vi "Demo_Copy.vi"() -> ()   [LabVIEW 2018]
uses:
  <vilib>/Hampel Software Engineering/S7NetCom/Source/Controls/S7_Start_Address.ctl
  <vilib>/Hampel Software Engineering/S7NetCom/Source/Controls/S7_Memory_Area.ctl
  <vilib>/Hampel Software Engineering/S7NetCom/Source/Controls/S7_Variable_Type.ctl
  <vilib>/Hampel Software Engineering/S7NetCom/Source/API/Write Data - Boolean (Scalar).vi
  <vilib>/Hampel Software Engineering/S7NetCom/Source/API/Write Data - String.vi
  <vilib>/Hampel Software Engineering/S7NetCom/Source/API/Write Data - DTL (Scalar).vi
  <vilib>/Hampel Software Engineering/S7NetCom/Source/API/Write Data - Siemens Date & Time (Scalar).vi
  <vilib>/Hampel Software Engineering/S7NetCom/Source/API/Write Data - Byte (Scalar).vi
  <vilib>/Hampel Software Engineering/S7NetCom/Source/API/Write Data - Word (Scalar).vi
  <vilib>/Hampel Software Engineering/S7NetCom/Source/API/Write Data - Real (Scalar).vi
  <vilib>/Hampel Software Engineering/S7NetCom/Source/API/Write Data - Real (1D Array).vi
  <vilib>/Hampel Software Engineering/S7NetCom/Source/API/Read Data - Boolean (Scalar).vi
  <vilib>/Hampel Software Engineering/S7NetCom/Source/API/Read Data - String.vi
  <vilib>/Hampel Software Engineering/S7NetCom/Source/API/Read Data - DTL (Scalar).vi
  <vilib>/Hampel Software Engineering/S7NetCom/Source/API/Read Data - Siemens Date&Time (Scalar).vi
  <vilib>/Hampel Software Engineering/S7NetCom/Source/API/Read Data - Byte (Scalar).vi
  <vilib>/Hampel Software Engineering/S7NetCom/Source/API/Read Data - Word (Scalar).vi
  <vilib>/Hampel Software Engineering/S7NetCom/Source/API/Read Data - Real (Scalar).vi
  <vilib>/Hampel Software Engineering/S7NetCom/Source/API/Read Data - Real (1D Array).vi
  <vilib>/Hampel Software Engineering/S7NetCom/Source/S7NetCom.lvclass
panel:
  out "time(ms)":u32
  in  "Tab Control TX":T1(tab)
  in  "TX Data":u32[](array[numeric])
  in  "Btn_WriteRaw":bool
  in  "Btn_WriteBOOL":bool
  in  "Boolean Value (TX)":bool
  out "Boolean Value (RX)":bool
  in  "Btn_ReadBOOL":bool
  in  "Btn_WriteBYTE":bool
  in  "Byte Value (TX)":u8
  out "Byte Value (RX)":u8
  in  "Btn_ReadBYTE":bool
  in  "Btn_WriteWORD":bool
  in  "Word Value (TX)":u16
  out "Word Value (RX)":u16
  in  "Btn_ReadWORD":bool
  in  "Btn_WriteREAL":bool
  in  "Real Value (TX)":sgl
  out "Real Value (RX)":sgl
  in  "Btn_ReadREAL":bool
  in  "Real Values (TX)":sgl[](array[numeric])
  in  "Btn_WriteREALArray":bool
  in  "Btn_ReadREALArray":bool
  out "Real Values (RX)":sgl[](array[numeric])
  in  "String Read Length":u16
  out "String Value (RX)":string
  in  "String Value (TX)":string
  in  "Btn_WriteSTRING":bool
  in  "Btn_ReadSTRING":bool
  in  "Btn_ReadDTL":bool
  out "DTL Value (RX)":timestamp
  in  "DTL (TX)":timestamp
  in  "Btn_Write DTL":bool
  in  "Date & Time (TX)":timestamp
  in  "Btn_Write D&T":bool
  in  "Btn_ReadD&T":bool
  out "Date&Time Value (RX)":timestamp
  in  "stop":bool
  in  "Count":u16=1 caption="Read Length"
  in  "Start Address":T2
  in  "Data Block #":u16=2
  in  "RAW Var Type":T3=enum."BYTE"
  in  "Memory Area":T4=132 items=["P Area"=128, "I Area"=129, "O Area"=130, "M Area"=131, "DB Area"=132, "Counter"=40, "Timer"=41]
  in  "Bit Offset":u8
  out "Read/Write Error out":errorcluster
  out "U32":i32[](array[numeric])
  out "String":string
  out "Char's":string[](array[string])
  out "Bits (1st byte)":bool[](array[boolean])
  in  "Cont Variable Type":T3=enum."BYTE" caption="Variable Type"
  in  "Cont Memory Area":T4=132 caption="Memory Area" items=["P Area"=128, "I Area"=129, "O Area"=130, "M Area"=131, "DB Area"=132, "Counter"=40, "Timer"=41]
  in  "Cont Start Address":T2 caption="Start Address"
  in  "Cont Read Length":u16=1 caption="Read Length"
  in  "Cont Data Block #":u16=2 caption="Data Block #"
  out "Real (32bit)":sgl
  in  "Cont Bit Offset":u8 caption="Bit Offset"
  out "Seq No":u16
  in  "Cont TO":i32=250
  in  "Rack":u8
  out "Error out":errorcluster caption="Read Continuously Error out"
  in  "IP Address":string
  in  "Port":i32=102
  in  "Slot":u8=1
  in  "Timeout":i32=5000
  # "Connection"
  # "Read Continuously"
  # "Read / Write"
  # "说明：感谢该组织开源库，\n本VI为拷贝自S7NetCom库，通过安装S7NetCom.vip可在安装目录获取该范例。\n粗略测试，一次最多读230个字节，低延时。"
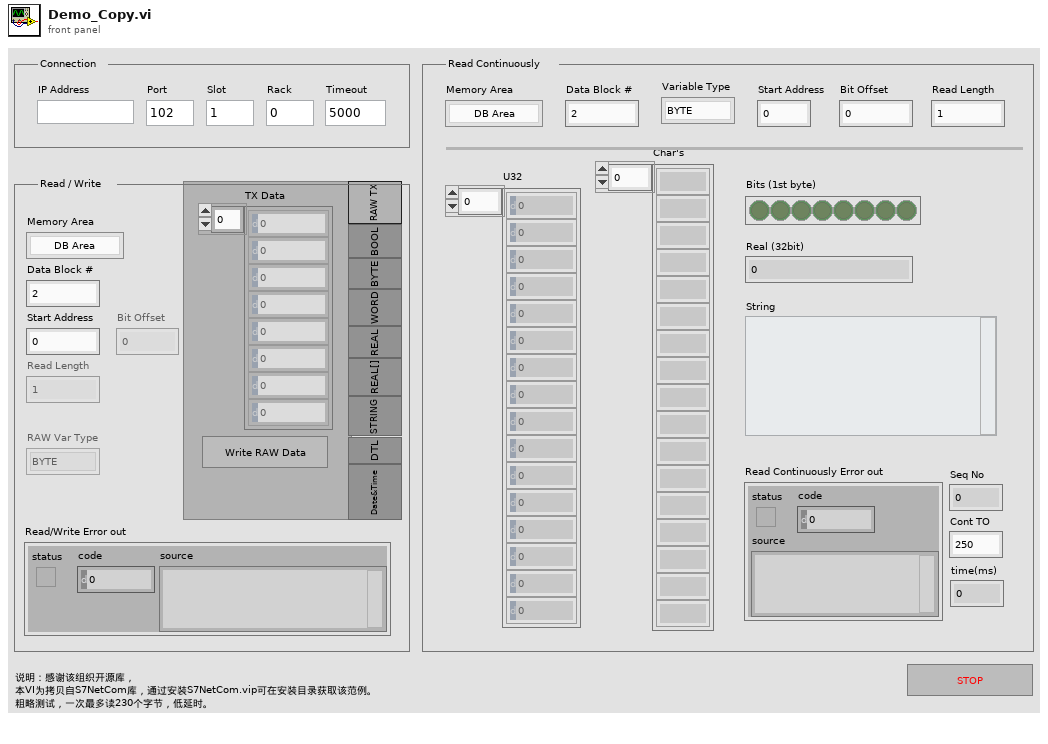
[diagram p1: front panel]
types:
  T1 = enum32{"RAW TX", "BOOL", "BYTE", "WORD", "REAL", "REAL[]", "STRING", "DTL", "Date&Time"}
  T2 = typedef "S7NetCom.lvlib/S7NetCom.lvclass/S7_Start_Address.ctl" = u32
  T3 = typedef "S7NetCom.lvlib/S7NetCom.lvclass/S7_Variable_Type.ctl" = enum8{"---", "BIT", "BYTE", "CHAR", "WORD", "INT", "DWORD", "DINT", "REAL"}
  T4 = typedef "S7NetCom.lvlib/S7NetCom.lvclass/S7_Memory_Area.ctl" = u8
  T5 = enum8{"Enabled", "Disabled", "Disabled and Grayed Out"}
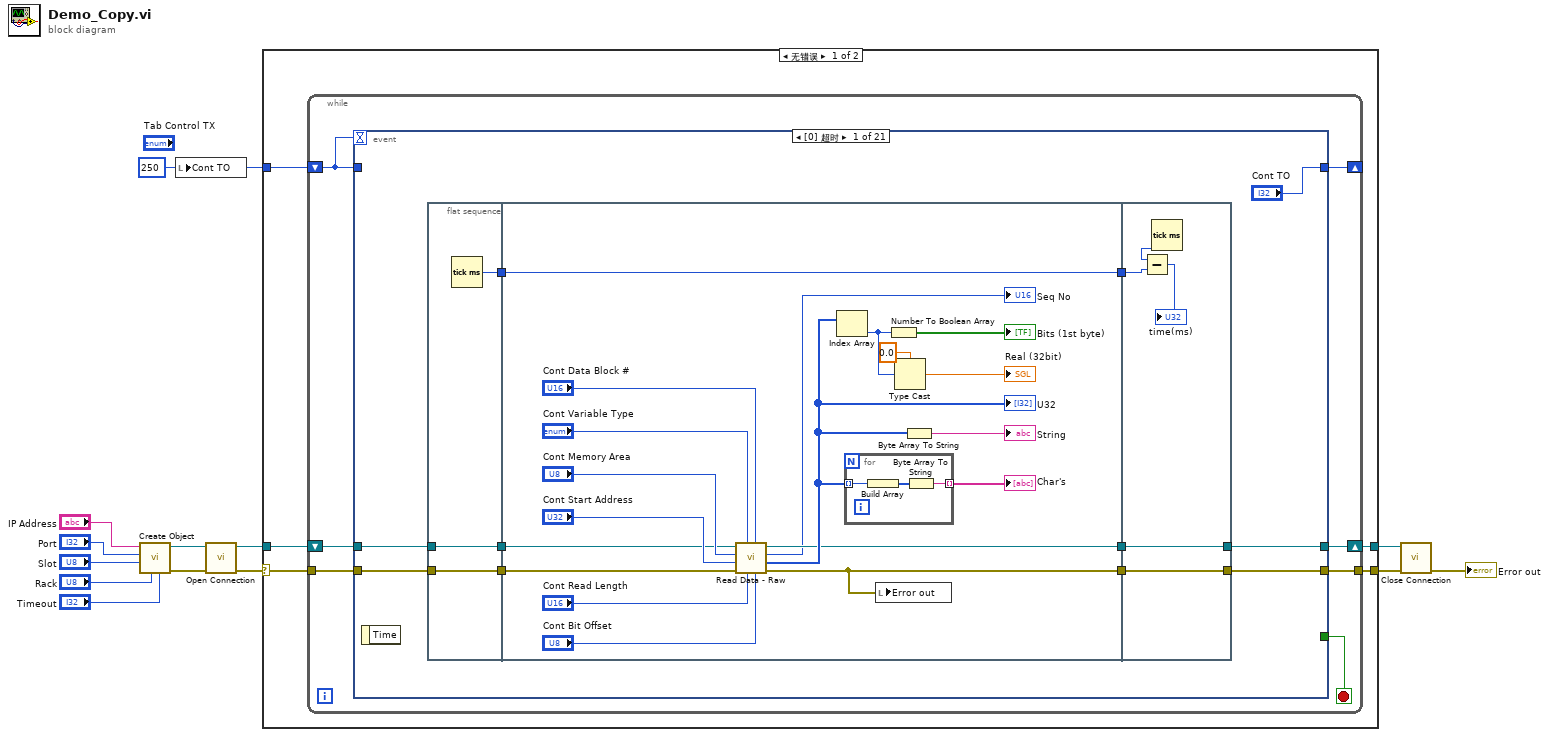
[diagram p0: block diagram]
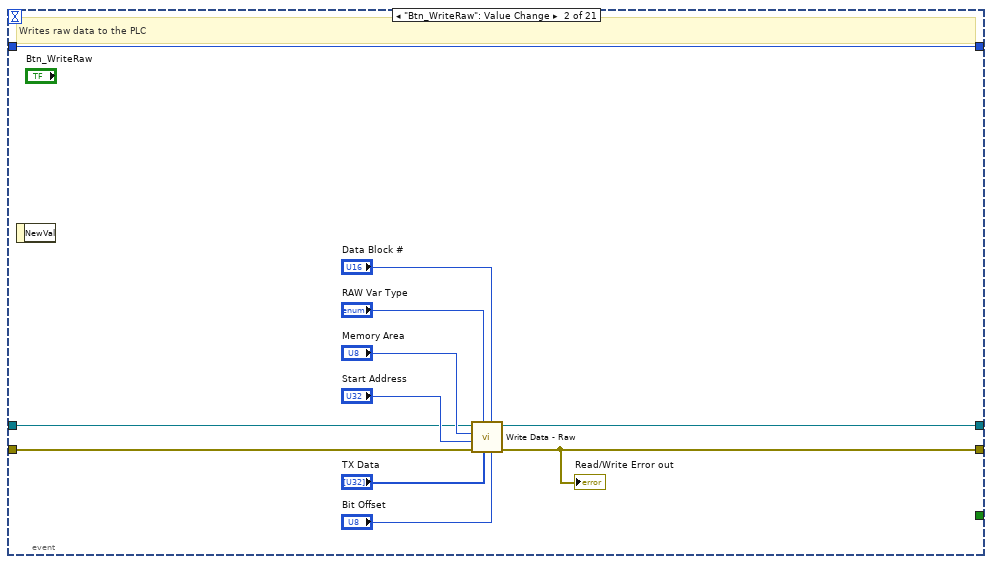
[diagram p2: hidden frame]
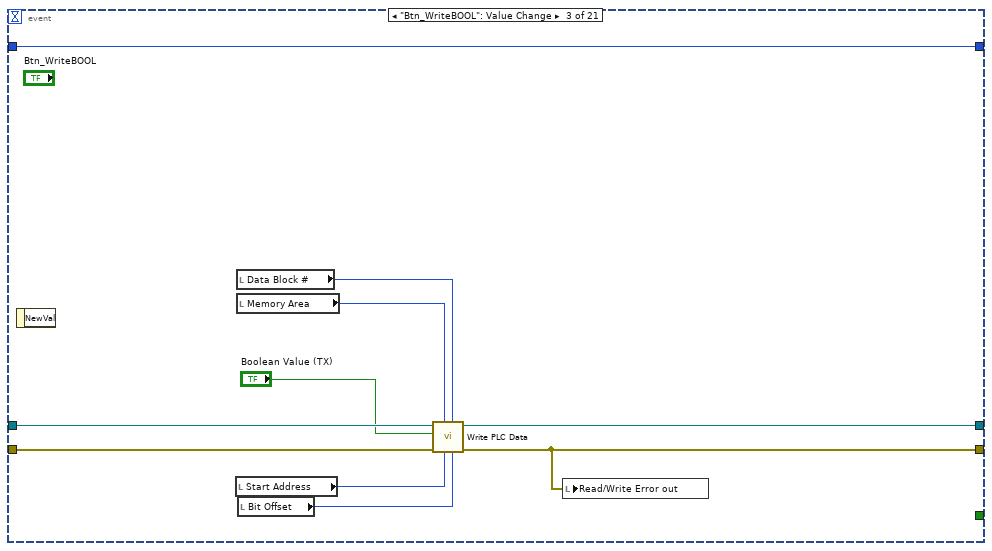
[diagram p3: hidden frame]
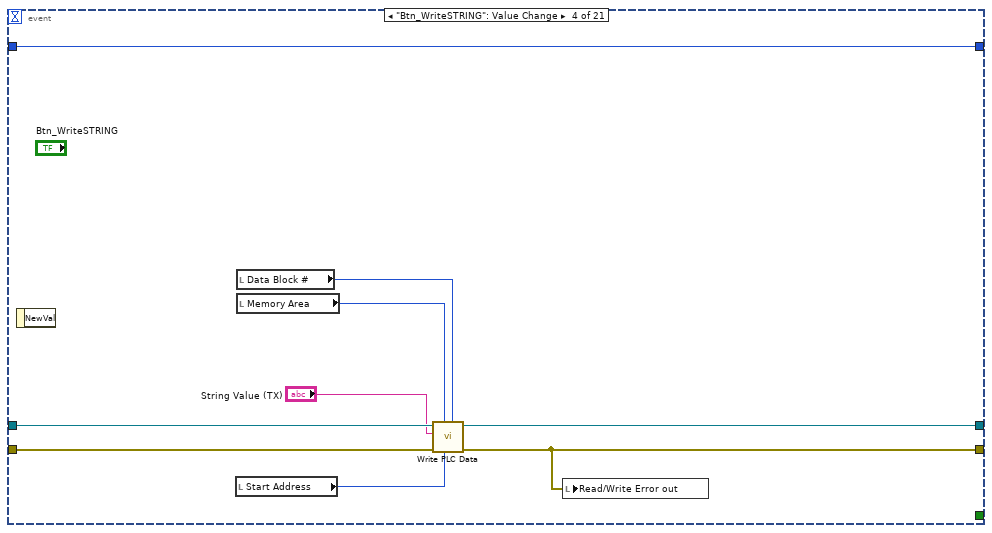
[diagram p4: hidden frame]
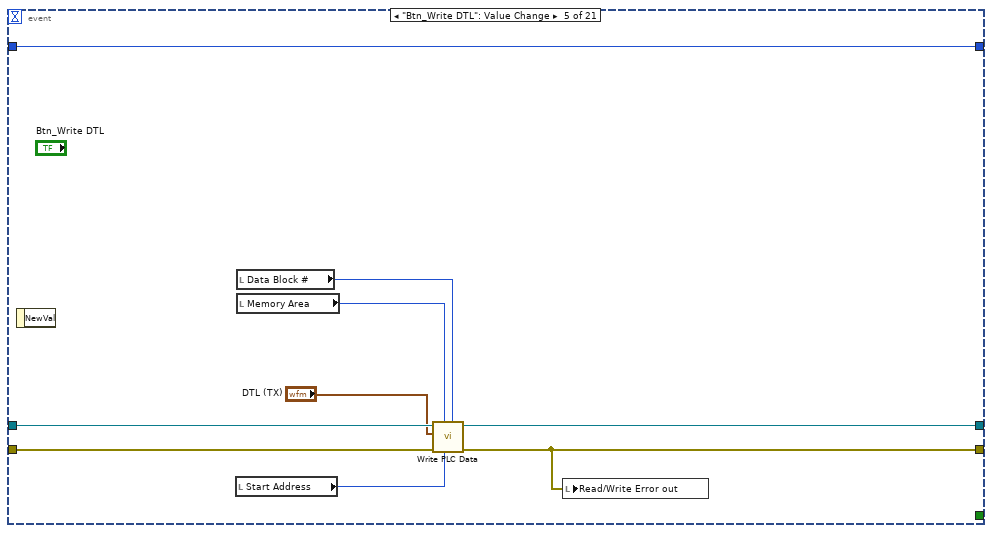
[diagram p5: hidden frame]
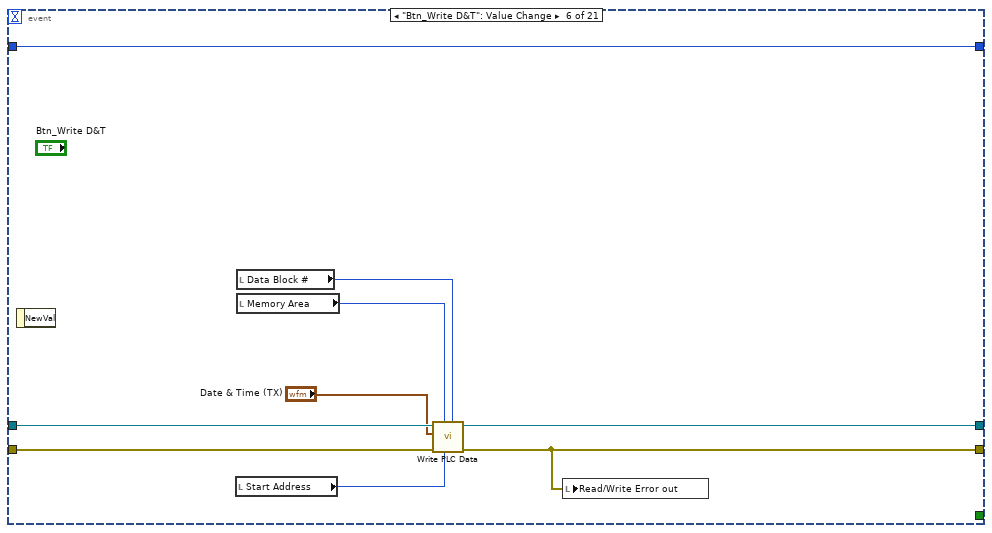
[diagram p6: hidden frame]
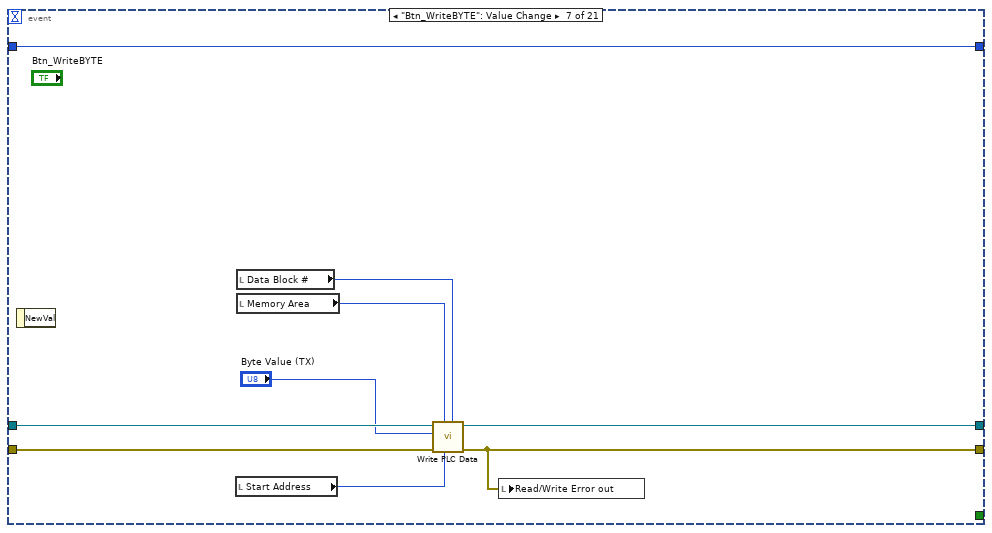
[diagram p7: hidden frame]
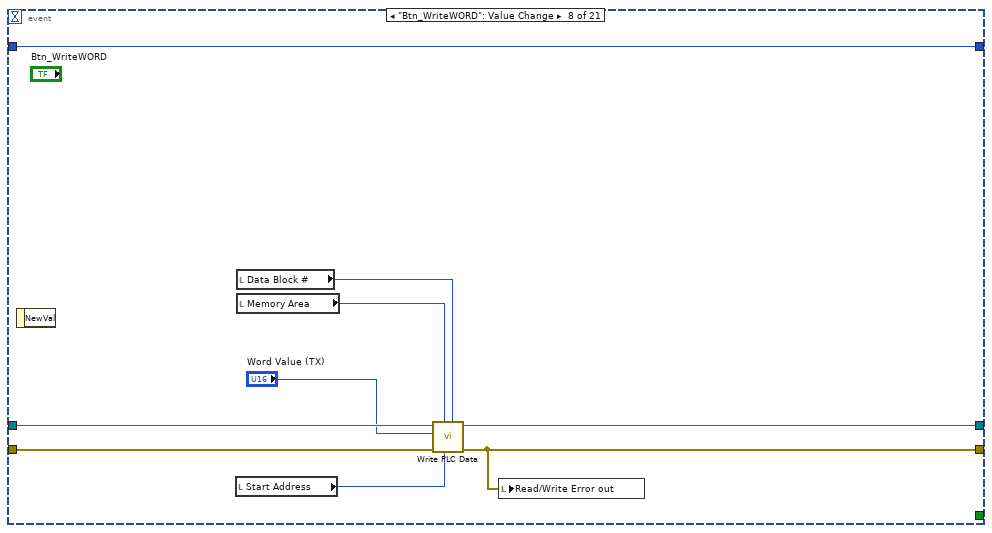
[diagram p8: hidden frame]
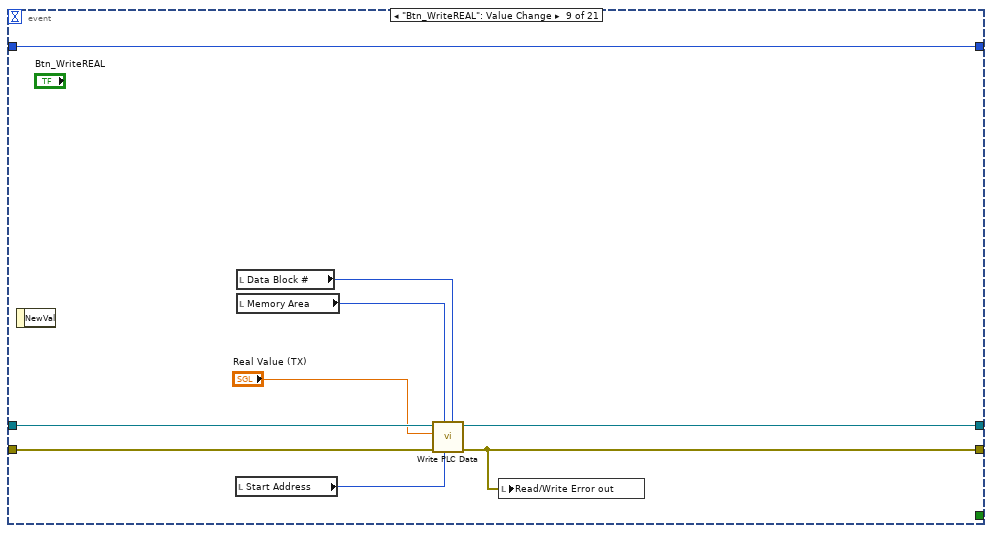
[diagram p9: hidden frame]
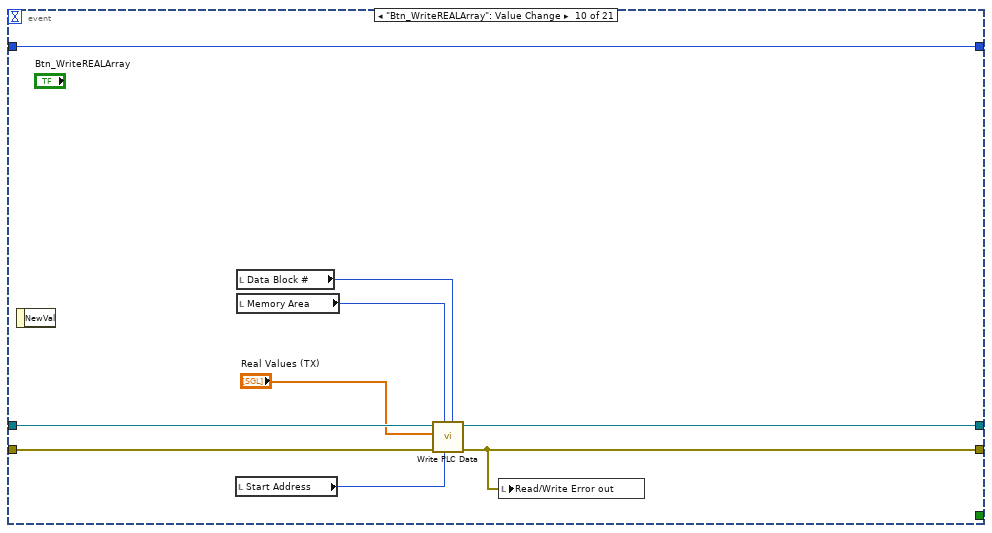
[diagram p10: hidden frame]
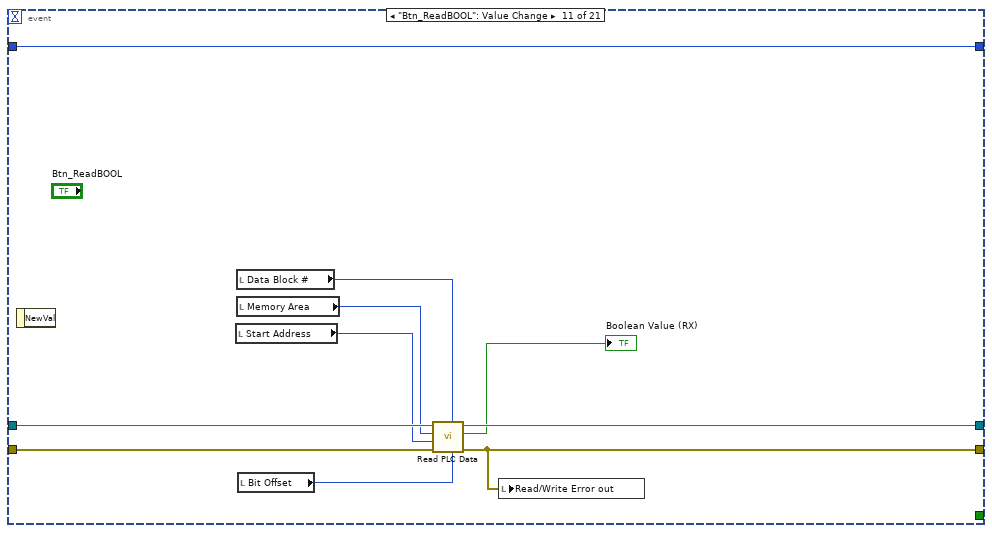
[diagram p11: hidden frame]
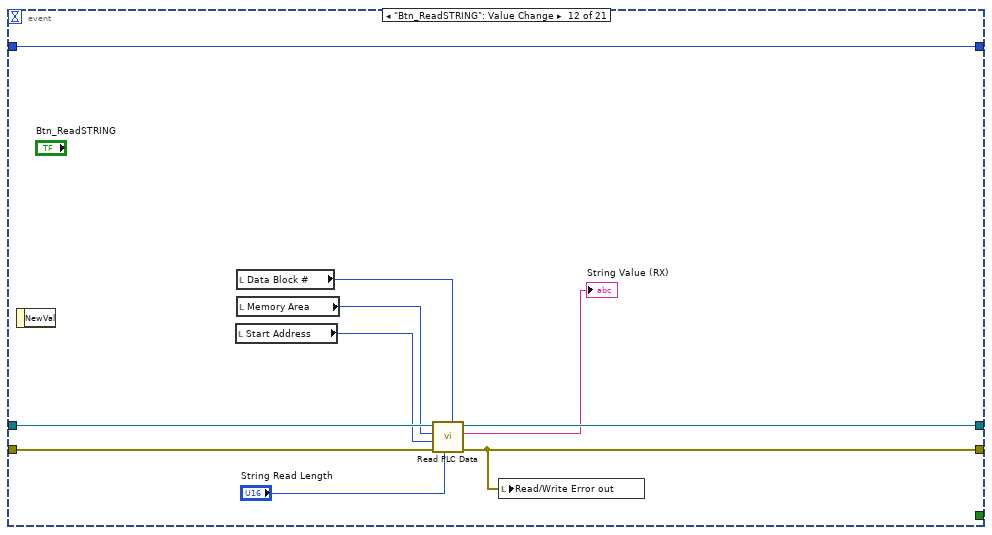
[diagram p12: hidden frame]
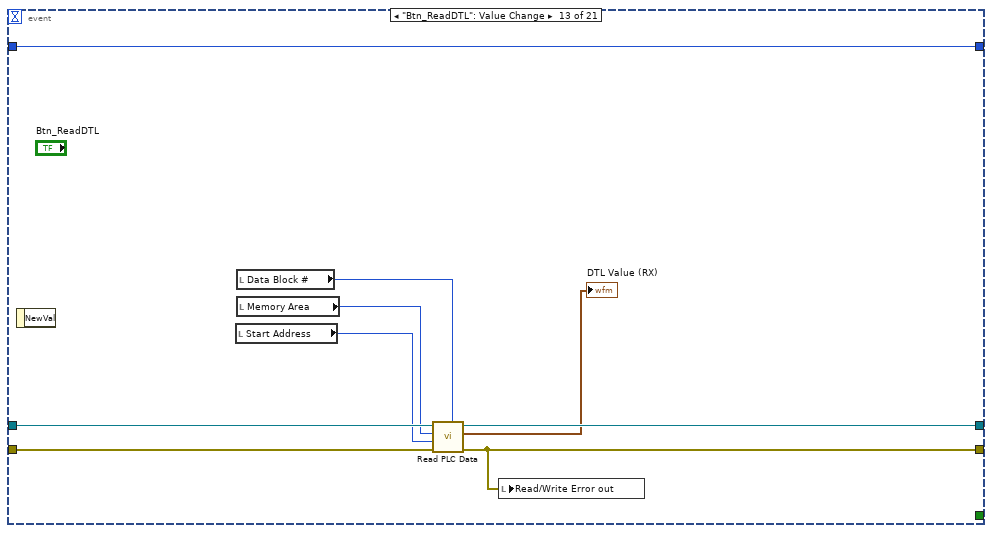
[diagram p13: hidden frame]
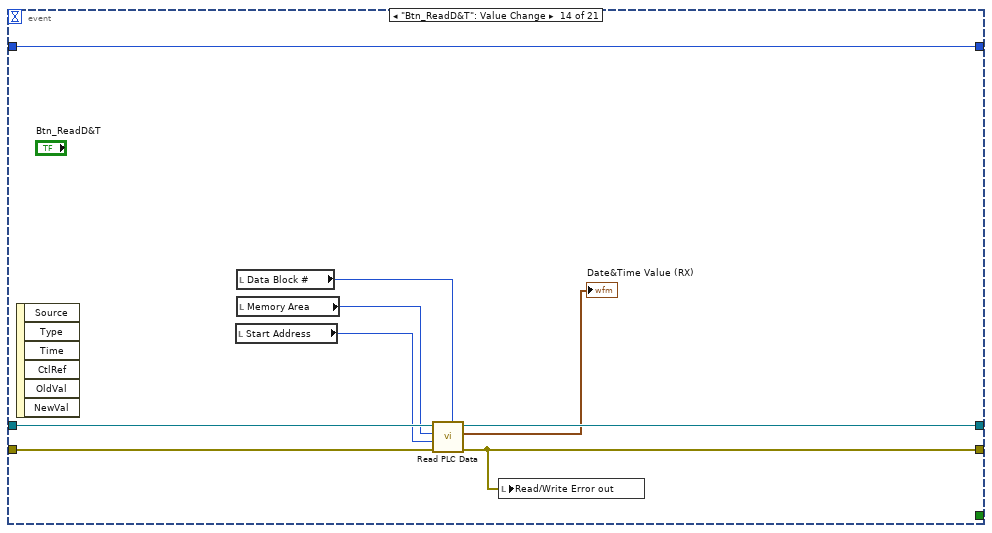
[diagram p14: hidden frame]
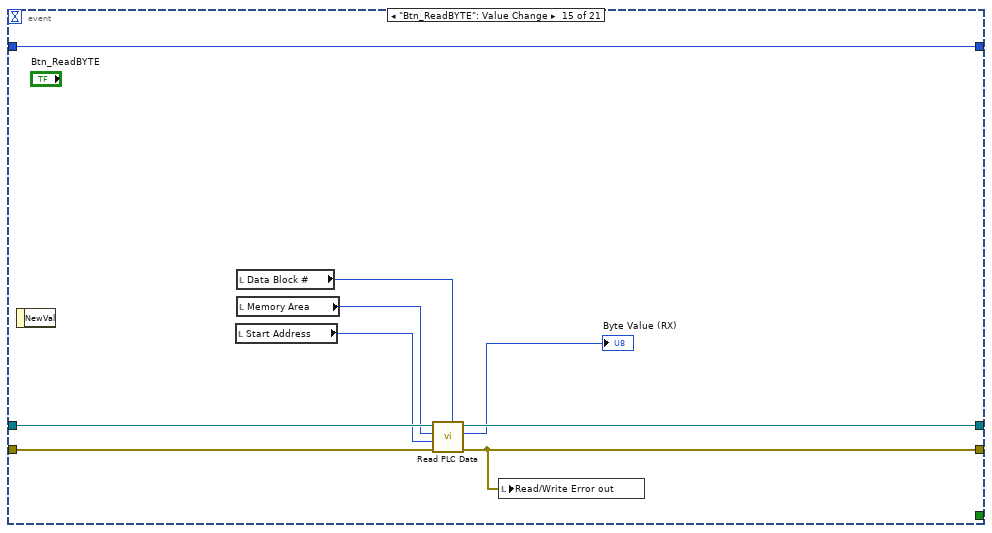
[diagram p15: hidden frame]
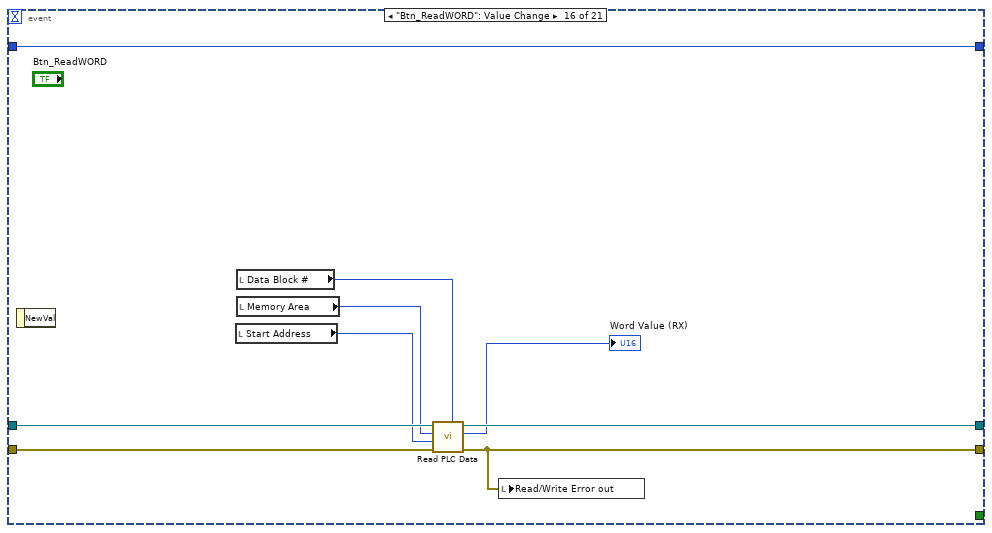
[diagram p16: hidden frame]
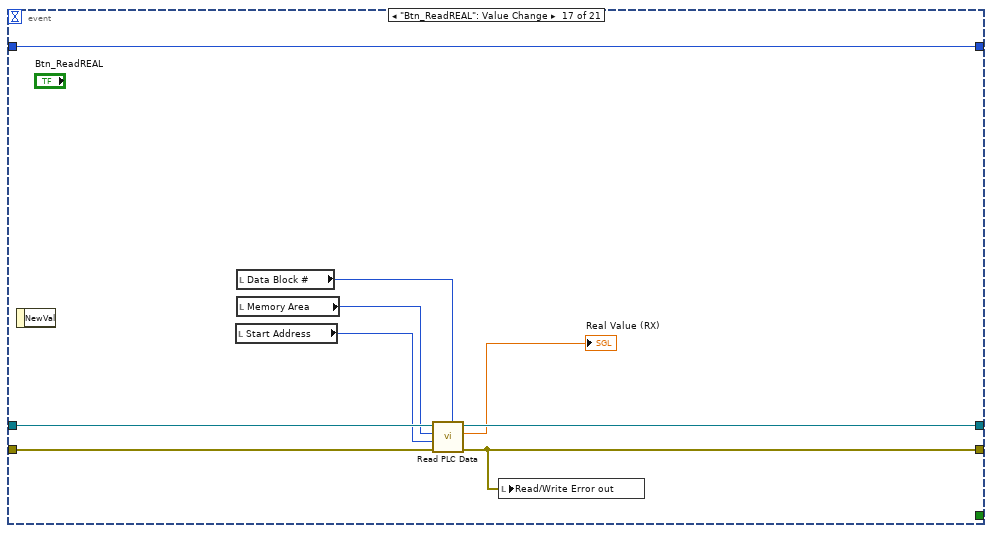
[diagram p17: hidden frame]
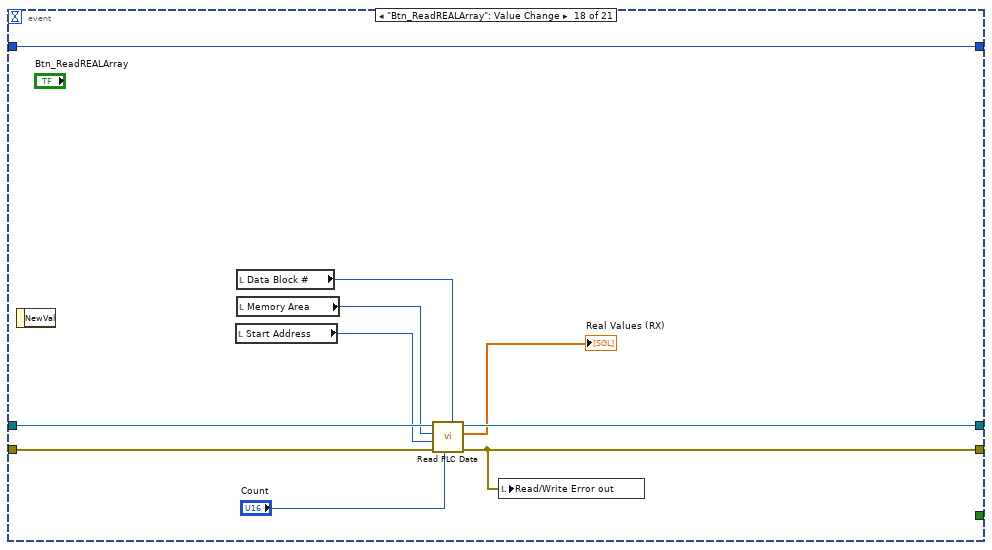
[diagram p18: hidden frame]
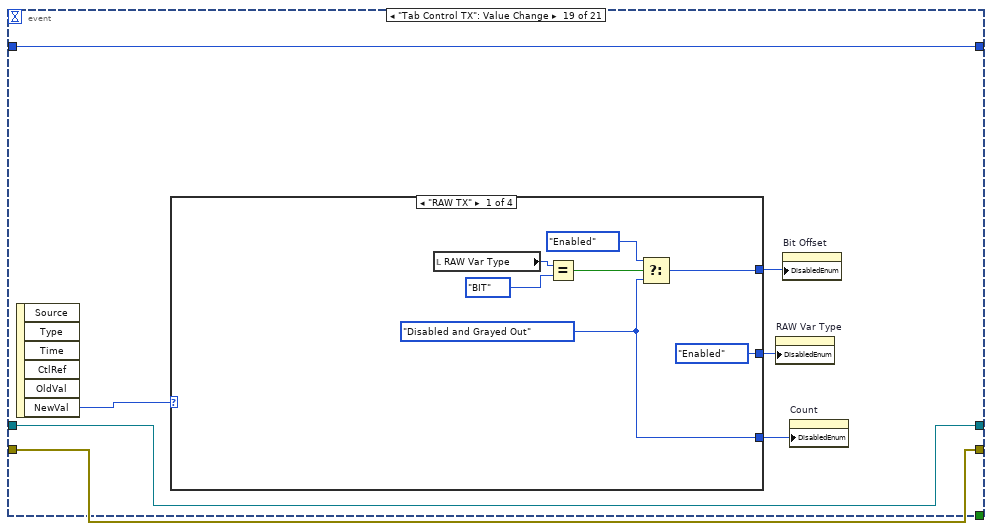
[diagram p19: hidden frame]
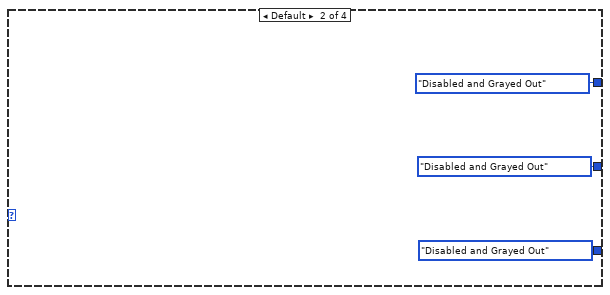
[diagram p20: hidden frame]
diagram:
  w1 = 250
  n1 = call <vilib>:"Create Object.vi"("Timeout"="Timeout", "Rack"="Rack", "Slot"="Slot", "Port"="Port", "IP Address"="IP Address") -> ("error out"=w10:errorcluster, "S7NetCom out"=w13:refnum<class "S7NetCom.lvclass">)  [unwired: 5 in]
  n2 = local write "Cont TO"(w1) -> ()
  n3 = call <vilib>:"Open Connection.vi"("error in"=w10, "S7NetCom in"=w13) -> ("error out"=w9:errorcluster, "S7NetCom out"=w12:refnum<class "S7NetCom.lvclass">)  [unwired: 8 in]
  n4 = case shown="无错误" w9 {
    selector: w9 -> [w15 w259]
    tunnel: w12 -> [w18 w260]
    tunnel: [w17 w260] -> w11
    tunnel: [w16 w259] -> w8
    tunnel: w1 -> [w14 _]
    frame No Error {
      n5 = while {
        shift-right: [w23] -> w17
        shift-left: w18 -> [w25]
        tunnel: [w21] -> w16
        tunnel: w15 -> [w22]
        shift-right: [w19] -> _
        shift-left: w14 -> [w20]
        stop <- w24 stop-if-true
        n6 = event shown="[0] 超时" {
          selector: _ -> [_ _ _ _ _ _ _ _ _ _ _ _ _ _ _ _ _ _ _ _ _]
          dyn-events: _ -> [_ _ _ _ _ _ _ _ _ _ _ _ _ _ _ _ _ _ _ _ _]
          timeout: w20 -> [_ _ _ _ _ _ _ _ _ _ _ _ _ _ _ _ _ _ _ _ _]
          tunnel: w25 -> [w36 w70 w86 w95 w104 w113 w122 w131 w140 w149 w159 w169 w178 w187 w196 w205 w214 w224 w226 w250 w257]
          tunnel: [_ _ _ _ _ _ _ _ _ _ _ _ _ _ _ _ _ _ _ _ w258] -> w24
          tunnel: [w35 w69 w84 w93 w102 w111 w120 w129 w138 w147 w157 w167 w176 w185 w194 w203 w212 w222 w226 w250 w257] -> w23
          tunnel: w22 -> [w33 w71 w87 w96 w105 w114 w123 w132 w141 w150 w160 w170 w179 w188 w197 w206 w215 w225 w227 w251 w256]
          tunnel: [w34 w68 w85 w94 w103 w112 w121 w130 w139 w148 w158 w168 w177 w186 w195 w204 w213 w223 w227 w251 w256] -> w21
          tunnel: w20 -> [_ w67 w78 w89 w98 w107 w115 w124 w133 w142 w151 w163 w172 w181 w189 w198 w207 w216 w232 w252 w255]
          tunnel: ["Cont TO" w67 w78 w89 w98 w107 w115 w124 w133 w142 w151 w163 w172 w181 w189 w198 w207 w216 w232 w252 w255] -> w19
          event Timeout {
            n7 = event-data() -> ()  [unwired: 1 in, 1 out]
            n8 = flat-sequence {
              tunnel: w33 -> [w38]
              tunnel: w36 -> [w39]
              tunnel: [w39] -> w31
              tunnel: [w38] -> w30
              tunnel: [w37] -> w27
              tunnel: w31 -> [w46]
              tunnel: w30 -> [w43]
              tunnel: [w45] -> w29
              tunnel: [w44] -> w28
              tunnel: w27 -> [w40]
              tunnel: [w40] -> w26
              tunnel: [w65] -> w34
              tunnel: [w66] -> w35
              tunnel: w29 -> [w66]
              tunnel: w28 -> [w65]
              tunnel: w26 -> [w63]
              frame #0 {
                n9 = Tick Count (ms)() -> (millisecond timer value=w37:u32)
              }
              frame #1 {
                n10 = call <vilib>:"Read Data - Raw.vi"("Bit Offset"="Cont Bit Offset", "Data Block #"="Cont Data Block #", "Read Length"="Cont Read Length", "Variable Type"="Cont Variable Type", "error in (no error)"=w43, "Start Address"="Cont Start Address", "Memory Area"="Cont Memory Area", "S7 in"=w46) -> ("error out"=w44:errorcluster, "Read Data"=w50:i32[], "Sequence No"=→"Seq No":u16, "S7 out"=w45:refnum<class "S7NetCom.lvclass">)
                "U32" <- w50
                n11 = Index Array(array=w50) -> (element=w49:i32)  [unwired: 1 in]
                n12 = for {
                  tunnel: w50 -> [w61] mode=indexing
                  tunnel: [w60] -> w57 mode=indexing
                  n13 = Build Array(w61) -> (w59:i32[])
                  n14 = Byte Array To String(unsigned byte array=w59) -> (string=w60:string)
                }
                "Char's" <- w57
                n15 = local write "Error out"(w44) -> ()
                n16 = Number To Boolean Array(number=w49) -> (Boolean array=→"Bits (1st byte)":bool[])
                n17 = Type Cast(type=sgl 0.0 ("Real (32bit)"), x=w49) -> (*(type *) &x=→"Real (32bit)":sgl)
                n18 = Byte Array To String(unsigned byte array=w50) -> (string=→"String":string)
              }
              frame #2 {
                n19 = Tick Count (ms)() -> (millisecond timer value=w64:u32)
                n20 = Subtract(x=w64, y=w63) -> (x-y=→"time(ms)":u32)
              }
            }
          }
          event "Btn_WriteRaw": Value Change {
            # "Writes raw data to the PLC"
            n21 = event-data() -> ()  [unwired: 1 in, 1 out]
            n22 = call <vilib>:"Write Data - Raw.vi"("Bit Offset"="Bit Offset", "Data Block #"="Data Block #", "Write Data"="TX Data", "Variable Type"="RAW Var Type", "error in (no error)"=w71, "Start Address"="Start Address", "Memory Area"="Memory Area", "S7 in"=w70) -> ("error out"=w68:errorcluster, "S7 out"=w69:refnum<class "S7NetCom.lvclass">)  [unwired: 2 in]
            "Read/Write Error out" <- w68
          }
          event "Btn_WriteBOOL": Value Change {
            n23 = event-data() -> ()  [unwired: 1 in, 1 out]
            n24 = local read "Start Address"() -> (w81:T2)
            n25 = local read "Data Block #"() -> (w83:u16)
            n26 = local read "Memory Area"() -> (w80:T4)
            n27 = local read "Bit Offset"() -> (w82:u8)
            n28 = call-poly <vilib>:"Write PLC Data.vi"("Bit Offset"=w82, "Data Block #"=w83, "Start Address"=w81, "Memory Area"=w80, "error in (no error)"=w87, "Value"="Boolean Value (TX)", "S7 in"=w86) -> ("error out"=w85:errorcluster, "S7 out"=w84:refnum<class "S7NetCom.lvclass">)  [unwired: 3 in]
            n29 = local write "Read/Write Error out"(w85) -> ()
          }
          event "Btn_WriteSTRING": Value Change {
            n30 = event-data() -> ()  [unwired: 1 in, 1 out]
            n31 = local read "Start Address"() -> (w91:T2)
            n32 = local read "Data Block #"() -> (w92:u16)
            n33 = local read "Memory Area"() -> (w90:T4)
            n34 = call-poly <vilib>:"Write PLC Data.vi"("Data Block #"=w92, "Start Address"=w91, "Memory Area"=w90, "error in (no error)"=w96, "String"="String Value (TX)", "S7 in"=w95) -> ("error out"=w94:errorcluster, "S7 out"=w93:refnum<class "S7NetCom.lvclass">)  [unwired: 4 in]
            n35 = local write "Read/Write Error out"(w94) -> ()
          }
          event "Btn_Write DTL": Value Change {
            n36 = event-data() -> ()  [unwired: 1 in, 1 out]
            n37 = local read "Start Address"() -> (w100:T2)
            n38 = local read "Data Block #"() -> (w101:u16)
            n39 = local read "Memory Area"() -> (w99:T4)
            n40 = call-poly <vilib>:"Write PLC Data.vi"("Data Block #"=w101, "Start Address"=w100, "Memory Area"=w99, "error in (no error)"=w105, "Value"="DTL (TX)", "S7 in"=w104) -> ("error out"=w103:errorcluster, "S7 out"=w102:refnum<class "S7NetCom.lvclass">)  [unwired: 4 in]
            n41 = local write "Read/Write Error out"(w103) -> ()
          }
          event "Btn_Write D&T": Value Change {
            n42 = event-data() -> ()  [unwired: 1 in, 1 out]
            n43 = local read "Start Address"() -> (w109:T2)
            n44 = local read "Data Block #"() -> (w110:u16)
            n45 = local read "Memory Area"() -> (w108:T4)
            n46 = call-poly <vilib>:"Write PLC Data.vi"("Data Block #"=w110, "Start Address"=w109, "Memory Area"=w108, "error in (no error)"=w114, "Value"="Date & Time (TX)", "S7 in"=w113) -> ("error out"=w112:errorcluster, "S7 out"=w111:refnum<class "S7NetCom.lvclass">)  [unwired: 4 in]
            n47 = local write "Read/Write Error out"(w112) -> ()
          }
          event "Btn_WriteBYTE": Value Change {
            n48 = event-data() -> ()  [unwired: 1 in, 1 out]
            n49 = local read "Start Address"() -> (w117:T2)
            n50 = local read "Data Block #"() -> (w118:u16)
            n51 = local read "Memory Area"() -> (w119:T4)
            n52 = call-poly <vilib>:"Write PLC Data.vi"("Data Block #"=w118, "Start Address"=w117, "Memory Area"=w119, "error in (no error)"=w123, "Value"="Byte Value (TX)", "S7 in"=w122) -> ("error out"=w121:errorcluster, "S7 out"=w120:refnum<class "S7NetCom.lvclass">)  [unwired: 4 in]
            n53 = local write "Read/Write Error out"(w121) -> ()
          }
          event "Btn_WriteWORD": Value Change {
            n54 = event-data() -> ()  [unwired: 1 in, 1 out]
            n55 = local read "Start Address"() -> (w126:T2)
            n56 = local read "Data Block #"() -> (w127:u16)
            n57 = local read "Memory Area"() -> (w128:T4)
            n58 = call-poly <vilib>:"Write PLC Data.vi"("Data Block #"=w127, "Start Address"=w126, "Memory Area"=w128, "error in (no error)"=w132, "Value"="Word Value (TX)", "S7 in"=w131) -> ("error out"=w130:errorcluster, "S7 out"=w129:refnum<class "S7NetCom.lvclass">)  [unwired: 4 in]
            n59 = local write "Read/Write Error out"(w130) -> ()
          }
          event "Btn_WriteREAL": Value Change {
            n60 = event-data() -> ()  [unwired: 1 in, 1 out]
            n61 = local read "Start Address"() -> (w135:T2)
            n62 = local read "Data Block #"() -> (w136:u16)
            n63 = local read "Memory Area"() -> (w137:T4)
            n64 = call-poly <vilib>:"Write PLC Data.vi"("Data Block #"=w136, "Start Address"=w135, "Memory Area"=w137, "error in (no error)"=w141, "Value"="Real Value (TX)", "S7 in"=w140) -> ("error out"=w139:errorcluster, "S7 out"=w138:refnum<class "S7NetCom.lvclass">)  [unwired: 4 in]
            n65 = local write "Read/Write Error out"(w139) -> ()
          }
          event "Btn_WriteREALArray": Value Change {
            n66 = event-data() -> ()  [unwired: 1 in, 1 out]
            n67 = local read "Start Address"() -> (w144:T2)
            n68 = local read "Data Block #"() -> (w145:u16)
            n69 = local read "Memory Area"() -> (w146:T4)
            n70 = call-poly <vilib>:"Write PLC Data.vi"("Data Block #"=w145, "Start Address"=w144, "Memory Area"=w146, "error in (no error)"=w150, "Values"="Real Values (TX)", "S7 in"=w149) -> ("error out"=w148:errorcluster, "S7 out"=w147:refnum<class "S7NetCom.lvclass">)  [unwired: 4 in]
            n71 = local write "Read/Write Error out"(w148) -> ()
          }
          event "Btn_ReadBOOL": Value Change {
            n72 = event-data() -> ()  [unwired: 1 in, 1 out]
            n73 = local read "Start Address"() -> (w154:T2)
            n74 = local read "Data Block #"() -> (w155:u16)
            n75 = local read "Memory Area"() -> (w156:T4)
            n76 = local read "Bit Offset"() -> (w152:u8)
            n77 = call-poly <vilib>:"Read PLC Data.vi"("Bit Offset"=w152, "Data Block #"=w155, "error in (no error)"=w160, "Start Address"=w154, "Memory Area"=w156, "S7 in"=w159) -> ("error out"=w158:errorcluster, "Boolean Value"=→"Boolean Value (RX)":bool, "S7 out"=w157:refnum<class "S7NetCom.lvclass">)  [unwired: 3 in]
            n78 = local write "Read/Write Error out"(w158) -> ()
          }
          event "Btn_ReadSTRING": Value Change {
            n79 = event-data() -> ()  [unwired: 1 in, 1 out]
            n80 = local read "Start Address"() -> (w164:T2)
            n81 = local read "Data Block #"() -> (w165:u16)
            n82 = local read "Memory Area"() -> (w166:T4)
            n83 = call-poly <vilib>:"Read PLC Data.vi"("Data Block #"=w165, "Read Length"="String Read Length", "error in (no error)"=w170, "Start Address"=w164, "Memory Area"=w166, "S7 in"=w169) -> ("error out"=w168:errorcluster, "String Value"=→"String Value (RX)":string, "S7 out"=w167:refnum<class "S7NetCom.lvclass">)  [unwired: 3 in]
            n84 = local write "Read/Write Error out"(w168) -> ()
          }
          event "Btn_ReadDTL": Value Change {
            n85 = event-data() -> ()  [unwired: 1 in, 1 out]
            n86 = local read "Start Address"() -> (w173:T2)
            n87 = local read "Data Block #"() -> (w174:u16)
            n88 = local read "Memory Area"() -> (w175:T4)
            n89 = call-poly <vilib>:"Read PLC Data.vi"("Data Block #"=w174, "error in (no error)"=w179, "Start Address"=w173, "Memory Area"=w175, "S7 in"=w178) -> ("error out"=w177:errorcluster, "Time Stamp"=→"DTL Value (RX)":timestamp, "S7 out"=w176:refnum<class "S7NetCom.lvclass">)  [unwired: 4 in]
            n90 = local write "Read/Write Error out"(w177) -> ()
          }
          event "Btn_ReadD&T": Value Change {
            n91 = event-data() -> ()  [unwired: 1 in, 6 out]
            n92 = local read "Start Address"() -> (w182:T2)
            n93 = local read "Data Block #"() -> (w183:u16)
            n94 = local read "Memory Area"() -> (w184:T4)
            n95 = call-poly <vilib>:"Read PLC Data.vi"("Data Block #"=w183, "error in (no error)"=w188, "Start Address"=w182, "Memory Area"=w184, "S7 in"=w187) -> ("error out"=w186:errorcluster, "Time Stamp"=→"Date&Time Value (RX)":timestamp, "S7 out"=w185:refnum<class "S7NetCom.lvclass">)  [unwired: 4 in]
            n96 = local write "Read/Write Error out"(w186) -> ()
          }
          event "Btn_ReadBYTE": Value Change {
            n97 = event-data() -> ()  [unwired: 1 in, 1 out]
            n98 = local read "Start Address"() -> (w191:T2)
            n99 = local read "Data Block #"() -> (w192:u16)
            n100 = local read "Memory Area"() -> (w193:T4)
            n101 = call-poly <vilib>:"Read PLC Data.vi"("Data Block #"=w192, "error in (no error)"=w197, "Start Address"=w191, "Memory Area"=w193, "S7 in"=w196) -> ("error out"=w195:errorcluster, "Byte Value"=→"Byte Value (RX)":u8, "S7 out"=w194:refnum<class "S7NetCom.lvclass">)  [unwired: 4 in]
            n102 = local write "Read/Write Error out"(w195) -> ()
          }
          event "Btn_ReadWORD": Value Change {
            n103 = event-data() -> ()  [unwired: 1 in, 1 out]
            n104 = local read "Start Address"() -> (w200:T2)
            n105 = local read "Data Block #"() -> (w201:u16)
            n106 = local read "Memory Area"() -> (w202:T4)
            n107 = call-poly <vilib>:"Read PLC Data.vi"("Data Block #"=w201, "error in (no error)"=w206, "Start Address"=w200, "Memory Area"=w202, "S7 in"=w205) -> ("error out"=w204:errorcluster, "Word Value"=→"Word Value (RX)":u16, "S7 out"=w203:refnum<class "S7NetCom.lvclass">)  [unwired: 4 in]
            n108 = local write "Read/Write Error out"(w204) -> ()
          }
          event "Btn_ReadREAL": Value Change {
            n109 = event-data() -> ()  [unwired: 1 in, 1 out]
            n110 = local read "Start Address"() -> (w209:T2)
            n111 = local read "Data Block #"() -> (w210:u16)
            n112 = local read "Memory Area"() -> (w211:T4)
            n113 = call-poly <vilib>:"Read PLC Data.vi"("Data Block #"=w210, "error in (no error)"=w215, "Start Address"=w209, "Memory Area"=w211, "S7 in"=w214) -> ("error out"=w213:errorcluster, "Real Value"=→"Real Value (RX)":sgl, "S7 out"=w212:refnum<class "S7NetCom.lvclass">)  [unwired: 4 in]
            n114 = local write "Read/Write Error out"(w213) -> ()
          }
          event "Btn_ReadREALArray": Value Change {
            n115 = event-data() -> ()  [unwired: 1 in, 1 out]
            n116 = local read "Start Address"() -> (w218:T2)
            n117 = local read "Data Block #"() -> (w220:u16)
            n118 = local read "Memory Area"() -> (w221:T4)
            n119 = call-poly <vilib>:"Read PLC Data.vi"("Data Block #"=w220, "Count"="Count", "error in (no error)"=w225, "Start Address"=w218, "Memory Area"=w221, "S7 in"=w224) -> ("error out"=w223:errorcluster, "Real Values"=→"Real Values (RX)":sgl[], "S7 out"=w222:refnum<class "S7NetCom.lvclass">)  [unwired: 3 in]
            n120 = local write "Read/Write Error out"(w223) -> ()
          }
          event "Tab Control TX": Value Change {
            n121 = event-data() -> ("NewVal"=w231:T1)  [unwired: 1 in, 5 out]
            n122 = case shown="\"RAW TX\"" w231 {
              tunnel: [w235 T5."Disabled and Grayed Out" ("Disabled") T5."Disabled and Grayed Out" ("Disabled") T5."Enabled" ("Disabled")] -> w230
              tunnel: [T5."Enabled" ("Disabled") T5."Disabled and Grayed Out" ("Disabled") T5."Disabled and Grayed Out" ("Disabled") w246] -> w229
              tunnel: [w233 T5."Disabled and Grayed Out" ("Disabled") T5."Enabled" ("Disabled") w246] -> w228
              frame "RAW TX" {
                w233 = T5."Disabled and Grayed Out" ("Disabled")
                n123 = local read "RAW Var Type"() -> (w239:T3)
                n124 = Equal?(x=w239, y=S7_Variable_Type."BIT") -> (x = y?=w237:bool)
                n125 = Select(t=T5."Enabled" ("Disabled"), s=w237, f=w233) -> (s? t:f=w235:T5)
              }
              frame Default {
              }
              frame "REAL[]" {
              }
              frame "BOOL" {
                w246 = T5."Disabled and Grayed Out" ("Disabled")
              }
            }
            n126 = property on="RAW Var Type" class="Enum (严格)"("DisabledEnum"=w229) -> ()  [unwired: 2 in, 2 out]
            n127 = property on="Bit Offset" class="DigNum (严格)"("DisabledEnum"=w230) -> ()  [unwired: 2 in, 2 out]
            n128 = property on="Count" class="DigNum (严格)"("DisabledEnum"=w228) -> ()  [unwired: 2 in, 2 out]
          }
          event Value Change {
            n129 = event-data() -> ("NewVal"=w249:T3)  [unwired: 1 in, 5 out]
            n130 = case shown="\"---\", 默认" w249 {
              tunnel: [T5."Disabled and Grayed Out" ("Disabled") T5."Enabled" ("Disabled")] -> w248
              frame "---", Default {
              }
              frame "BIT" {
              }
            }
            n131 = property on="Bit Offset" class="DigNum (严格)"("DisabledEnum"=w248) -> ()  [unwired: 2 in, 2 out]
          }
          event "stop": Value Change {
            n132 = event-data() -> ("NewVal"=w258:bool)  [unwired: 1 in]
          }
        }
      }
    }
    frame Error {
    }
  }
  n133 = call <vilib>:"Close Connection.vi"("error in (no error)"=w8, "S7NetCom in"=w11) -> ("error out"=→"Error out":errorcluster)  [unwired: 8 in, 1 out]
